vi "Remove Write Protection NVM.vi"(0 "Session Handle in":T1, 11 "error in (no error)":errorcluster) -> (4 "Session Handle out":T1, 15 "error out":errorcluster)   [LabVIEW 2015, in "PAS.lvclass"]
uses:
  PAS.lvclass
  Typedefs/Session Handle.ctl
panel:
  out "Whole Payload":u8[](array[numeric])
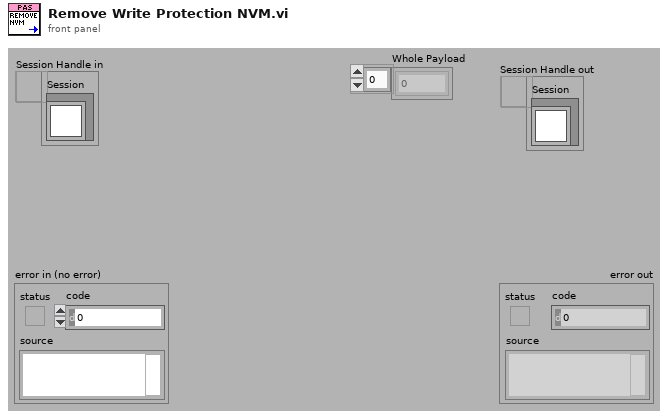
[diagram p1: front panel]
types:
  T1 = typedef "PAS.lvclass/Session Handle.ctl" = refnum<data-value>
  T2 = typedef "XNET Frame CAN.ctl" = cluster{"timestamp":timestamp, "payload":u8[], "identifier":u32, "type":T3, "extended?":bool, "echo?":bool}
  T3 = typedef "XNET Frame Type CAN.ctl" = u8
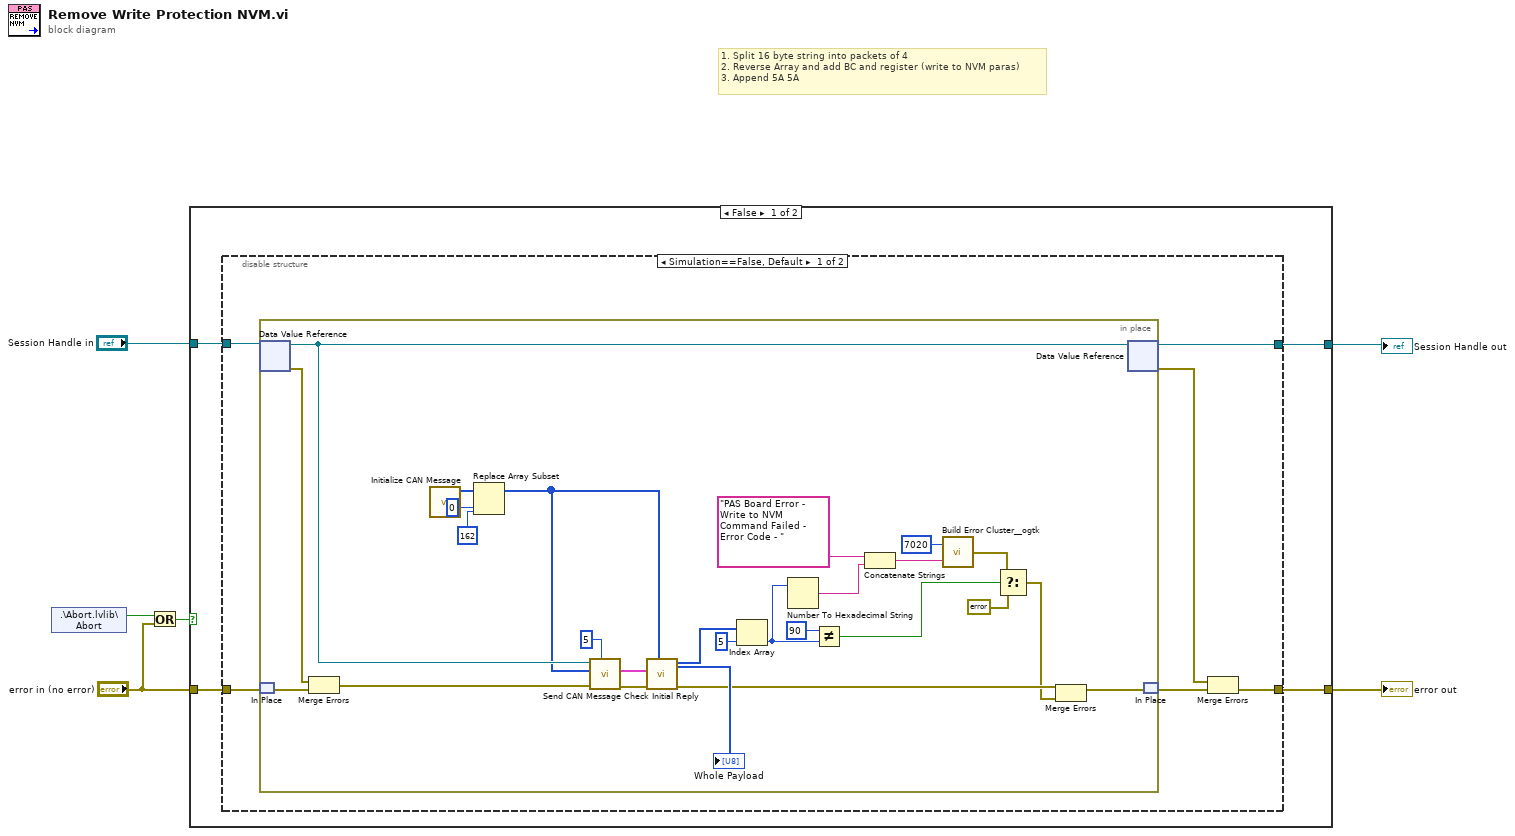
[diagram p0: block diagram]
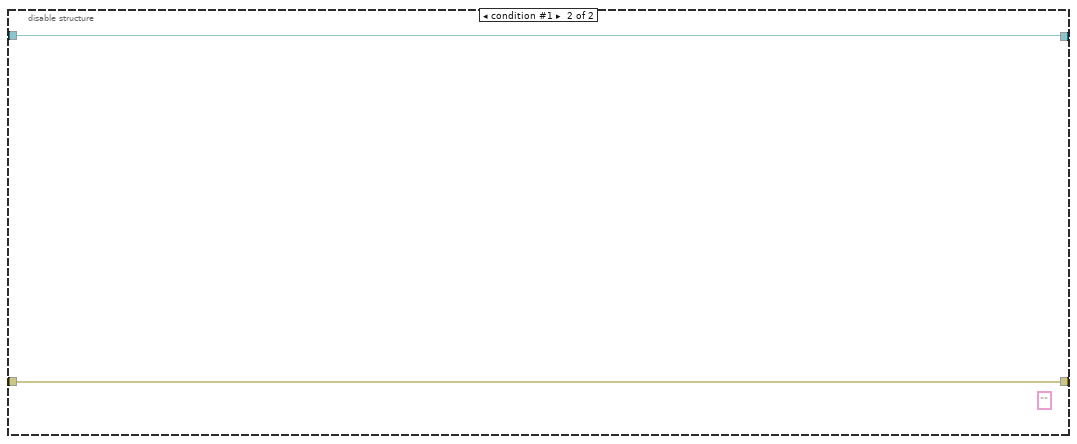
[diagram p2: hidden frame]
diagram:
  # "1. Split 16 byte string into packets of 4\n2. Reverse Array and add BC and register (write to NVM paras)\n3. Append 5A 5A"
  n1 = shared-variable ".\\Abort.lvlib\\Abort"() -> (w3:bool)  [unwired: 1 in, 1 out]
  n2 = Or(x=w3, y="error in (no error)") -> (x .or. y?=w1:bool)
  n3 = case shown="False" w1 {
    tunnel: [w10 w46] -> w5
    tunnel: [w9 w45] -> w4
    tunnel: "Session Handle in" -> [w8 w46]
    tunnel: "error in (no error)" -> [w7 w45]
    frame False {
      n4 = disable-structure shown="Simulation==False, Default" {
        disable-tunnel: [w16 w44] -> w10
        disable-tunnel: [w13 w43] -> w9
        disable-tunnel: w8 -> [w12 w44]
        disable-tunnel: w7 -> [w11 w43]
        frame condition #0 (active) {
          n5 = in-place {
            n6 = in-place-dvr #1(w12) -> (w39:refnum<class "PAS.lvclass">, w42:errorcluster)
            n7 = in-place-match #2(w11) -> (w41:errorcluster)
            n8 = Merge Errors(w42, w41) -> (w40:errorcluster)
            n9 = call "Initialize CAN Message.vi"() -> ("Initial Payload"=w20:u8[])  [unwired: 11 in]
            n10 = Replace Array Subset(array=w20, new element=u8 162 ("Numeric"), index=0) -> (w17:u8[])
            n11 = call "Send CAN Message.vi"("Number of Retries"=5, "error in (no error)"=w40, "payload"=w17, "Gas In"=w39) -> ("error out"=w23:errorcluster, "Reply"=w36:T2[])  [unwired: 5 in, 1 out]
            n12 = call "Check Initial Reply.vi"("Write Message"=w17, "error in (no error)"=w23, "Reply"=w36) -> ("error out"=w22:errorcluster, "Data Packet"=w32:u8[], "Whole Payload"=→"Whole Payload":u8[])  [unwired: 5 in, 1 out]
            n13 = Index Array(array=w32, index=5) -> (element=w28:u8)
            n14 = Number To Hexadecimal String(2:w28) -> (0:w27:string)  [unwired: 1 in]
            n15 = Not Equal?(x=u8 90, y=w28) -> (x != y?=w25:bool)
            n16 = Concatenate Strings("PAS Board Error - Write to NVM Command Failed - Error Code - " ("string"), w27) -> (w26:string)
            n17 = call <userlib>:"Build Error Cluster__ogtk.vi"("String to Prepend to source (\"\")"=w26, "code"=7020) -> ("error out"=w34:errorcluster)
            n18 = Select(t=w34, s=w25, f=errorcluster {"status"=FALSE, "code"=0, "source"=""}) -> (s? t:f=w21:errorcluster)
            n19 = Merge Errors(w22, w21) -> (w38:errorcluster)
            n20 = in-place-dvr #1(w39) -> (w16:T1, w14:errorcluster)
            n21 = in-place-match #2(w38) -> (w15:errorcluster)
          }
          n22 = Merge Errors(w14, w15) -> (w13:errorcluster)
        }
        frame condition #1 {
          (unwired) "" ("string")
        }
      }
    }
    frame True {
    }
  }
  "Session Handle out" <- w5
  "error out" <- w4
